vi "DAQmxTaskContainerFaradayCup-Com-Exec.vi"(8 "error in (no error)":errorcluster, 9 "data":variant, 10 "ControlQueue":refnum<queue>, 11 "DAQmxTaksContainer_General in":refnum<class "DAQmxTaksContainer_General.lvclass">) -> (0 "error out":errorcluster, 3 "DAQmxTaksContainer_General out":refnum<class "DAQmxTaksContainer_General.lvclass">)   [LabVIEW 2020, in "DAQmxTaksContainer_General.lvclass"]
uses:
  DAQmxTaksContainer_General.lvclass
  dependecies/ControlsVIs/Clusters-def/ProtypeCommand-DAQmxReply.ctl
  dependecies/ControlsVIs/Clusters-def/SERVER-Commands.ctl
  DAQmxTask.lvclass
  Control/Control-Server/Control-Server.lvclass
  dependecies/ControlsVIs/Clusters-def/Message types.ctl
  GeneralFunctionality/GeneralFunctionality.lvclass
  Message/Message.lvclass
  C:/dev/TRANCON/Classes/GeneralFunctionality/GeneralFunctionality.lvclass
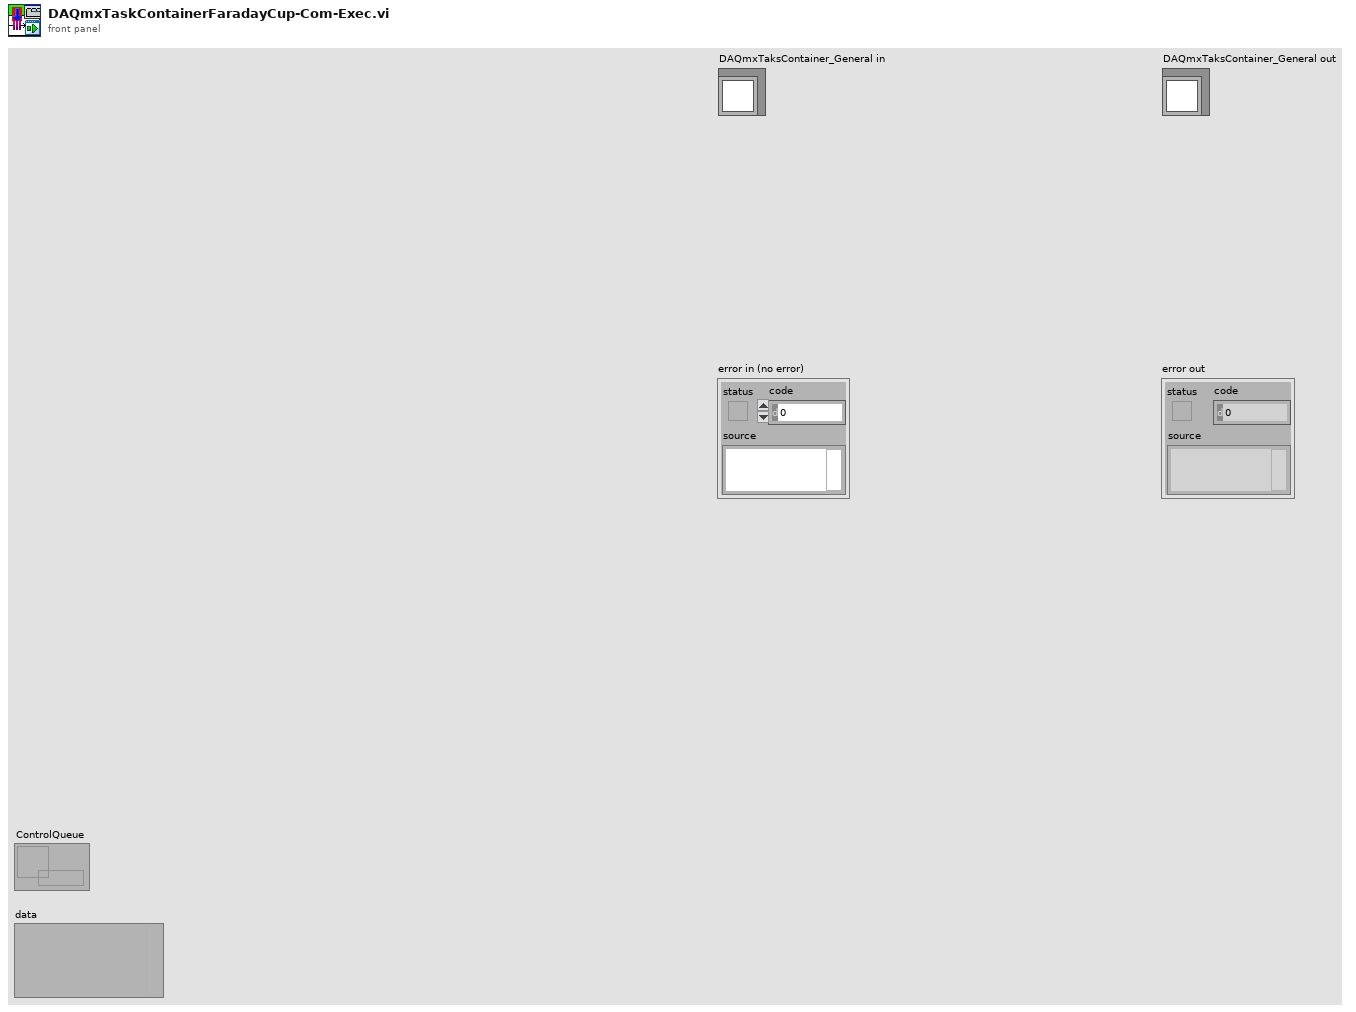
[diagram p1: front panel]
types:
  T1 = typedef "Control-Server.lvclass/SERVER-Commands.ctl" = string
  T2 = typedef "ProtypeCommand-DAQmxReply.ctl" = cluster{"On/Off":bool, "error out":errorcluster}
  T3 = typedef "Message types.ctl" = string
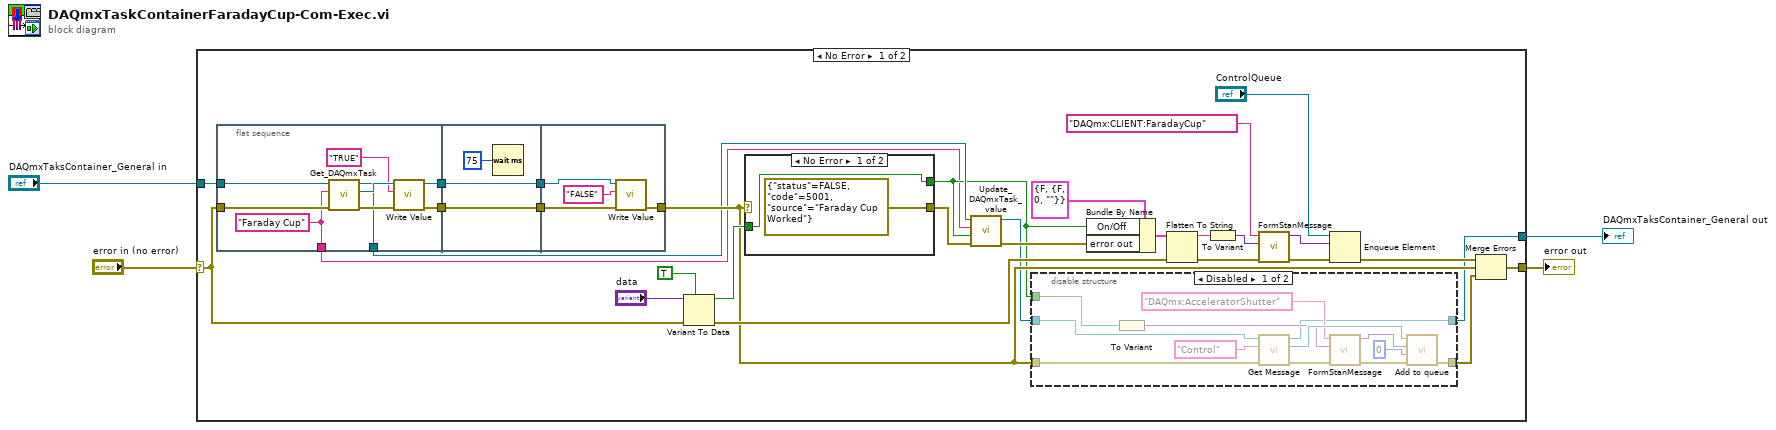
[diagram p0: block diagram]
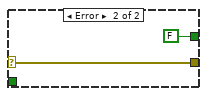
[diagram p3: hidden frame]
diagram:
  n1 = case shown="No Error" "error in (no error)" {
    selector: "error in (no error)" -> [w31 w71]
    tunnel: [w9 w70] -> w1
    tunnel: "DAQmxTaksContainer_General in" -> [w14 w70]
    tunnel: [w33 w71] -> w2
    frame No Error {
      n2 = flat-sequence {
        tunnel: w14 -> [w58]
        tunnel: w31 -> [w57]
        tunnel: [w53] -> w23
        tunnel: [w52] -> w21
        tunnel: [w51] -> w8
        tunnel: [w50] -> w5
        tunnel: w23 -> [w61]
        tunnel: [w61] -> w22
        tunnel: w21 -> [w59]
        tunnel: [w59] -> w20
        tunnel: [w64] -> w13
        tunnel: w22 -> [w65]
        tunnel: w20 -> [w62]
        frame #0 {
          w50 = "Faraday Cup" ("Task name")
          n3 = call "Get_DAQmxTask.vi"("error in (no error)"=w57, "Task name"=w50, "DAQmxTaksContainer_General in"=w58) -> ("error out"=w56:errorcluster, "DAQmx Task"=w55:refnum<class "DAQmxTask.lvclass">, "DAQmxTaksContainer_General out"=w51:refnum<class "DAQmxTaksContainer_General.lvclass">)  [unwired: 6 in]
          n4 = call-dynamic "Write Value.vi"("error in (no error)"=w56, "Data"="TRUE", "DAQmxTask en entrée"=w55) -> ("error out"=w53:errorcluster, "DAQmxTask en sortie"=w52:refnum<class "DAQmxTask.lvclass">)  [unwired: 7 in]
        }
        frame #1 {
          n5 = Wait (ms)(milliseconds to wait=u32 75) -> ()  [unwired: 1 out]
        }
        frame #2 {
          n6 = call-dynamic "Write Value.vi"("error in (no error)"=w65, "Data"="FALSE", "DAQmxTask en entrée"=w62) -> ("error out"=w64:errorcluster)  [unwired: 7 in, 1 out]
        }
      }
      n7 = Variant To Data(error in=w31, type=TRUE, Variant="data") -> (data=w28:bool, error out=w25:errorcluster)
      n8 = case shown="No Error" w13 {
        selector: w13 -> [_ w69]
        tunnel: [errorcluster {"status"=FALSE, "code"=5001, "source"="Faraday Cup Worked"} ("error constant") w69] -> w11
        tunnel: [w66 FALSE] -> w6
        tunnel: w28 -> [w66 _]
        frame No Error {
        }
        frame Error {
        }
      }
      n9 = call "Update_DAQmxTask_value.vi"("error in (no error)"=w11, "Value"=w6, "Task name"=w5, "DAQmxTaksContainer_General in"=w8) -> ("error out"=w10:errorcluster, "DAQmxTaksContainer_General out"=w7:refnum<class "DAQmxTaksContainer_General.lvclass">)  [unwired: 6 in]
      n10 = disable-structure shown="Disabled" {
        disable-tunnel: w13 -> [w46 w48]
        disable-tunnel: [w40 w48] -> w12
        disable-tunnel: [w37 w49] -> w9
        disable-tunnel: w7 -> [w36 w49]
        disable-tunnel: w6 -> [w35 _]
        frame Disabled {
          n11 = To Variant(anything=w35) -> (Variant=w38:variant)
          n12 = call "Get Message.vi"("error in (no error)"=w46, "Message type"=T3 "Control", "GeneralFunctionality en entrée"=w36) -> ("error out"=w44:errorcluster, "Message.lvclass"=w45:refnum<class "Message.lvclass">, "GeneralFunctionality en sortie"=w37:refnum<class "DAQmxTaksContainer_General.lvclass">)  [unwired: 6 in]
          n13 = call "FormStanMessage.vi"("error in"=w44, "data"=w38, "Command"="DAQmx:AcceleratorShutter") -> ("error out"=w43:errorcluster, "message"=w42:variant)  [unwired: 7 in]
          n14 = call "Add to queue.vi"("error in (no error)"=w43, "timeout in ms (-1)"=0, "Data"=w42, "Message in"=w45) -> ("error out"=w40:errorcluster)  [unwired: 6 in, 1 out]
        }
        frame Enabled {
        }
      }
      n15 = Bundle By Name(cluster=T2 {"On/Off"=FALSE, "error out"={"status"=FALSE, "code"=0, "source"=""}} ("output cluster"), "On/Off"=w6, "error out"=w10) -> (w26:T2)
      n16 = Flatten To String(anything=w26, error in (no error)=w25) -> (data string=w27:string, error out=w17:errorcluster)  [unwired: 2 in, 1 out]
      n17 = To Variant(anything=w27) -> (Variant=w18:variant)
      n18 = call "FormStanMessage.vi"("error in"=w17, "data"=w18, "Command"=T1 "DAQmx:CLIENT:FaradayCup" ("Commands")) -> ("error out"=w16:errorcluster, "message"=w15:variant)  [unwired: 7 in]
      n19 = Enqueue Element(queue="ControlQueue", element=w15, error in (no error)=w16) -> (error out=w24:errorcluster)  [unwired: 1 in, 2 out]
      n20 = Merge Errors(w24, w13, w12) -> (w33:errorcluster)
    }
    frame Error {
    }
  }
  "error out" <- w2
  "DAQmxTaksContainer_General out" <- w1
